vi "Clean Up Actor.vi"(8 "error in (no error)":errorcluster, 11 "Mediated Asynchronous Actor in":refnum<class "Mediated Asynchronous Actor.lvclass">) -> (0 "error out":errorcluster, 3 "Mediated Asynchronous Actor out":refnum<class "Mediated Asynchronous Actor.lvclass">)   [LabVIEW 2016, in "Stream Mediator.lvlib" / "Mediated Asynchronous Actor.lvclass"]
doc: "--\nCopyright © 2017 Composed SystemsI All rights reserved.\n\nAuthor: Jon McBee <jon.mcbee@composed.io>\n\nThis library is provided \"AS IS\" ,WITHOUT WARRANTIES OR\nCONDITIONS OF ANY KIND, either express or implied.\n\nComposed Systems -- composed.io\n\nStream 0.0.1.1\nJon McBee - Composed Systems\nCopyright (c) 2017, Composed Systems"
uses:
  <userlib>/Composed Systems/Stream/Mediator/Classes/Mediated Asynchronous Actor/Mediated Asynchronous Actor.lvclass
  C:/Program Files (x86)/National Instruments/LabVIEW 2016/user.lib/Composed Systems/Stream/Mediator/Classes/Mediated Actor/Mediated Actor.lvclass
  <userlib>/Composed Systems/Stream/Mediator/Classes/Mediated Asynchronous Actor/Mediated Asynchronous Actor.lvclass/Mediated Asynchronous Actor.ctl
  <userlib>/Composed Systems/Stream/Mediator/Classes/Mediated Actor/Mediated Actor.lvclass
  <userlib>/Composed Systems/Stream/Mediator/Classes/Message Broker Interface/Message Broker Interface.lvclass
  <userlib>/Composed Systems/Stream/Mediator/Classes/Message Transport Queue/Message Transport Queue.lvclass
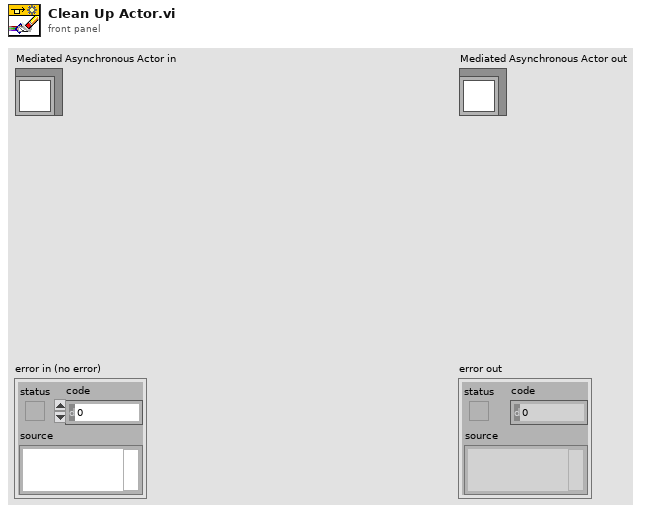
[diagram p1: front panel]
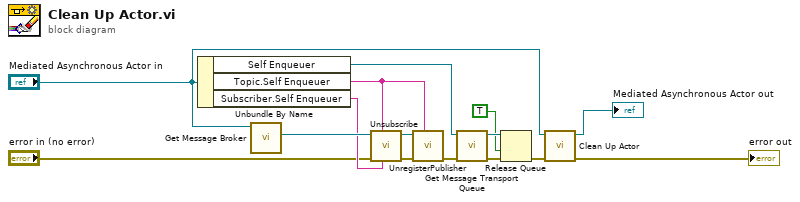
[diagram p0: block diagram]
diagram:
  n1 = Unbundle By Name("Mediated Asynchronous Actor in") -> ("Self Enqueuer"=w10:refnum<class "Message Transport Queue.lvclass">, "Topic.Self Enqueuer"=w1:string, "Subscriber.Self Enqueuer"=w7:string)
  n2 = call <userlib>:"Get Message Broker.vi"("Mediated Actor in"="Mediated Asynchronous Actor in") -> ("Message Broker"=w8:refnum<class "Message Broker Interface.lvclass">)  [unwired: 9 in, 1 out]
  n3 = call-dynamic "Unsubscribe.vi"("Subscriber Name"=w7, "Topic Name"=w1, "error in (no error)"="error in (no error)", "Message Broker Interface in"=w8) -> ("error out"=w9:errorcluster, "Message Broker Interface out"=w2:refnum<class "Message Broker Interface.lvclass">)  [unwired: 6 in]
  n4 = call-dynamic "UnregisterPublisher.vi"("Topic Name"=w1, "error in (no error)"=w9, "Message Broker Interface in"=w2) -> ("error out"=w3:errorcluster)  [unwired: 7 in, 1 out]
  n5 = call <userlib>:"Get Message Transport Queue.vi"("error in (no error)"=w3, "Message Transport Queue in"=w10) -> ("error out"=w13:errorcluster, "Queue"=w12:refnum<queue>)  [unwired: 8 in]
  n6 = Release Queue(queue=w12, force destroy? (F)=TRUE, error in (no error)=w13) -> (error out=w6:errorcluster)  [unwired: 2 out]
  n7 = call-parent "Clean Up Actor.vi"("error in (no error)"=w6, "Mediated Actor in"="Mediated Asynchronous Actor in") -> ("error out"=→"error out":errorcluster, "Mediated Actor out"=→"Mediated Asynchronous Actor out":refnum<class "Mediated Asynchronous Actor.lvclass">)  [unwired: 8 in]
